vi "SR430_read_bindata.vi"(0 "address":T1, 5 "error in (no error)":errorcluster) -> (14 "address out":T1, 16 "Data":u16[](array[numeric]), 17 "dataSum":u32, 19 "error out":errorcluster)   [LabVIEW 2009, in "SR430Driver.lvlib"]
doc: "Reads the entire display memory data record in binary format. \n\nCopyright (C)\nGesellschaft für Schwerionenforschung, GSI\nPlanckstr. 1\n64291 Darmstadt\nGermany\n\nContact: D.Beck@gsi.de \n\nThis program is free software; you can redistribute it and/or modify it under the terms of the \nGNU General Public License as published by the Free Software Foundation; either version 2 of the license, or (at your option) any later version.\n\nThis program is distributed in the hope that it will be useful, but WITHOUT ANY WARRANTY; without even the implied warranty of MERCHANTABILITY or FITNESS FOR A PARTICULAR PURPOSE. See the GNU General License for more details (http://www.gnu.org).\n\nGesellschaft für Schwerionenforschung, GSI\nPlanckstr. 1, 64291 Darmstadt, Germany\nFor all questions and ideas contact: M.Richter@gsi.de, K.Poppensieker, H.Brand@gsi.de or D.Beck@gsi.de.\nLast update: 11-APR-2002"
uses:
  SR430Driver.lvlib
  SR430_VISA Control.ctl
panel:
  # "SR430 Read Binary Data"
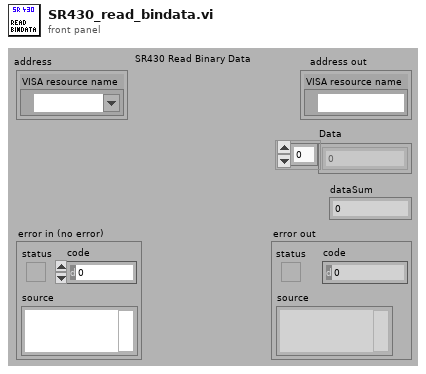
[diagram p1: front panel]
types:
  T1 = typedef "SR430Driver.lvlib/SR430_VISA Control.ctl" = cluster{"VISA resource name":refnum<visa-resource-name>}
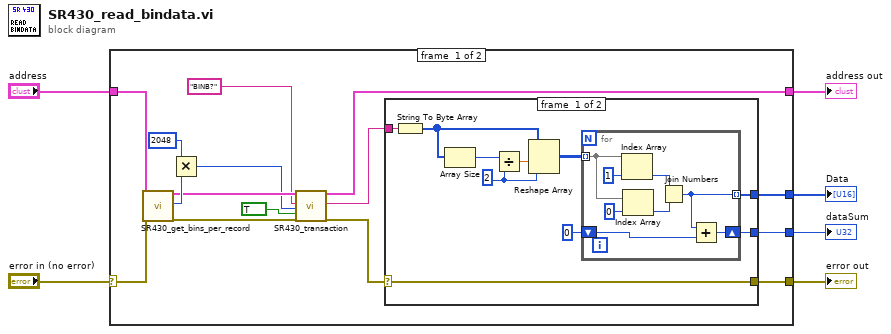
[diagram p0: block diagram]
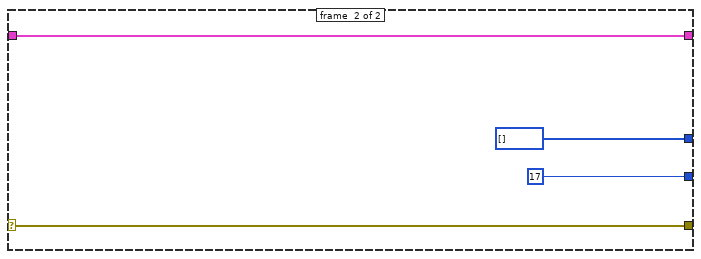
[diagram p3: hidden frame]
diagram:
  n1 = case shown="No Error" "error in (no error)" {
    selector: "error in (no error)" -> [w18 w42]
    tunnel: [w21 u16[] []] -> w6
    tunnel: "address" -> [w16 w41]
    tunnel: [w15 w42] -> w5
    tunnel: [w19 u16 17] -> w3
    tunnel: [w13 w41] -> w1
    frame #0 {
      n2 = call "SR430_get_bins_per_record.vi"("address"=w16, "error in (no error)"=w18) -> ("address out"=w14:T1, "binsPerRecord"=w17:i32, "error out"=w12:errorcluster)  [unwired: 15 in]
      n3 = Multiply(x=2048 ("byte count"), y=w17) -> (x*y=w7:i32)
      n4 = call "SR430_transaction.vi"("SR430 VISA Cluster"=w14, "SR430 Command String"="BINB?" ("write buffer"), "Bytes to read (1024)"=w7, "Read (FALSE)"=TRUE, "error in (no error)"=w12) -> ("dup SR430 VISA Cluster"=w13:T1, "SR430 Response"=w9:string, "error out"=w8:errorcluster)  [unwired: 11 in, 1 out]
      n5 = case shown="No Error" w8 {
        selector: w8 -> [w22 w40]
        tunnel: [w31 _] -> w21
        tunnel: [w30 _] -> w19
        tunnel: w9 -> [w29 _]
        tunnel: [w22 w40] -> w15
        frame #0 {
          w26 = 2 ("Dimension Size")
          n6 = String To Byte Array(string=w29) -> (unsigned byte array=w28:u8[])
          n7 = Array Size(array=w28) -> (size(s)=w27:i32)
          n8 = Divide(x=w27, y=w26) -> (x/y=w25:dbl)
          n9 = Reshape Array(w28, w25, w26) -> (w24:u8[][])
          n10 = for {
            tunnel: w24 -> [w39] mode=indexing
            tunnel: [w34] -> w31 mode=indexing
            shift-right: [w32] -> w30
            shift-left: u32 0 -> [w33]
            n11 = Index Array(array=w39, index=1 ("Index")) -> (element=w36:u8)
            n12 = Index Array(array=w39, index=0 ("Index")) -> (element=w35:u8)
            n13 = Join Numbers(hi=w36, lo=w35) -> ((hi.lo)=w34:u16)
            n14 = Add(x=w34, y=w33) -> (x+y=w32:u32)
          }
        }
        frame #1 {
        }
      }
    }
    frame #1 {
    }
  }
  "error out" <- w5
  "Data" <- w6
  "dataSum" <- w3
  "address out" <- w1
